vi "NiFPGA Write Array - I64.vi"(6 "Size":u32, 8 "error in (no error)":errorcluster, 9 "Array":i64[](array[numeric]), 10 "Control":u32, 11 "Session":u32) -> (0 "error out":errorcluster, 3 "Session Out":u32)   [LabVIEW 2010, in "FPGA Interface Wrapper.lvlib"]
doc: "Writes an entire array of signed 64-bit integer values to a given array control or indicator."
uses:
  <userlib>/_FPGA Interface Advanced Tools/FPGA Interface Wrapper/FPGA Interface Wrapper.lvlib
  NiFpga.dll
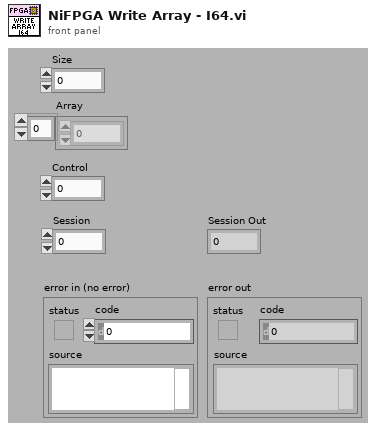
[diagram p1: front panel]
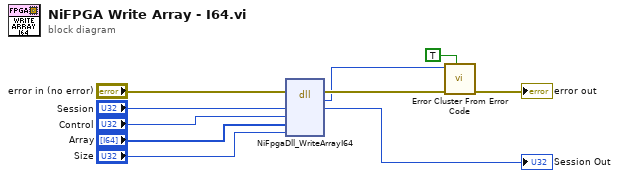
[diagram p0: block diagram]
diagram:
  n1 = dll-call lib="NiFpga.dll" fn="NiFpgaDll_WriteArrayI64"(error in="error in (no error)", "Session"="Session", "Control"="Control", "Array"="Array", "Size"="Size") -> (error out=w2:errorcluster, "Status"=w1:i32, "Session"=→"Session Out":u32)  [unwired: 5 in, 1 out]
  n2 = call <vilib>:"Error Cluster From Error Code.vi"("show call chain? (False)"=TRUE, "error in (no error)"=w2, "error code (0)"=w1) -> ("error out"=→"error out":errorcluster)  [unwired: 6 in]
